vi "DSF.Execution.Builder.Build.vi"(8 "error in (no error)":errorcluster, 9 "Transfer ID":i32, 10 "Plugin ID":i32, 11 "Builder in":refnum<class "DSF.Execution.Builder.lvclass">) -> (0 "error out":errorcluster, 3 "Builder out":refnum<class "DSF.Execution.Builder.lvclass">)   [LabVIEW 2016, in "DSF.Engine.lvlib" / "DSF.Execution.Builder.lvclass"]
uses:
  DSF.Execution.Builder.lvclass
  DSF.Execution.Builder.lvclass/DSF.Execution.Builder.ctl
  Memory.Cache/DSF.Memory.Cache.Framework.lvclass/DSF.Memory.Cache.Framework.ctl
  Memory.Cache/DSF.Memory.Cache.Plugin.lvclass/DSF.Memory.Cache.Plugin.ctl
  Memory.Cache/DSF.Memory.Cache.Transfer.lvclass/DSF.Memory.Cache.Transfer.ctl
  Memory.Pointer/DSF.Memory.Pointer.VS Channels.lvclass/DSF.Memory.Pointer.VS Channels.ctl
  Submodules/Memory Manager/Source/Classes/Pointer/Memory.Pointer.lvclass/Memory.Pointer.ctl
  Memory.Buffer/Methods/DSF.Memory.Buffer.Write.vi
  Memory.Buffer/Methods/DSF.Memory.Buffer.Write.1D.Bool.vi
  Memory.Buffer/Methods/DSF.Memory.Buffer.Write.1D.SGL.vi
  Memory.Buffer/Methods/DSF.Memory.Buffer.Write.1D.DBL.vi
  Memory.Buffer/Methods/DSF.Memory.Buffer.Write.1D.I8.vi
  Memory.Buffer/Methods/DSF.Memory.Buffer.Write.1D.I16.vi
  Memory.Buffer/Methods/DSF.Memory.Buffer.Write.1D.I32.vi
  Memory.Buffer/Methods/DSF.Memory.Buffer.Write.1D.I64.vi
  Memory.Buffer/Methods/DSF.Memory.Buffer.Write.1D.U8.vi
  Memory.Buffer/Methods/DSF.Memory.Buffer.Write.1D.U16.vi
  Memory.Buffer/Methods/DSF.Memory.Buffer.Write.1D.U32.vi
  Memory.Buffer/Methods/DSF.Memory.Buffer.Write.1D.U64.vi
  Memory.Cache/DSF.Memory.Cache.Framework.Get Plugin Caches.vi
  Memory.Cache/DSF.Memory.Cache.Plugin.Get Transfer Caches.vi
  Memory.Pointer/DSF.Memory.Pointer.VS Channels.Get Channel Count.vi
  Submodules/Memory Manager/Source/Classes/Pointer/Methods/Memory.Pointer.Read.vi
  Submodules/Memory Manager/Source/Classes/Pointer/Methods/Memory.Pointer.Read.Safe.1D.DBL.vi
  Submodules/Memory Manager/Source/Classes/Pointer/Methods/Memory.Pointer.Write.vi
  Submodules/Memory Manager/Source/Classes/Pointer/Methods/Memory.Pointer.Write.Safe.1D.Bool.vi
  Submodules/Memory Manager/Source/Classes/Pointer/Methods/Memory.Pointer.Write.Safe.1D.SGL.vi
  Submodules/Memory Manager/Source/Classes/Pointer/Methods/Memory.Pointer.Write.Safe.1D.DBL.vi
  Submodules/Memory Manager/Source/Classes/Pointer/Methods/Memory.Pointer.Write.Safe.1D.I8.vi
  Submodules/Memory Manager/Source/Classes/Pointer/Methods/Memory.Pointer.Write.Safe.1D.I16.vi
  Submodules/Memory Manager/Source/Classes/Pointer/Methods/Memory.Pointer.Write.Safe.1D.I32.vi
  Submodules/Memory Manager/Source/Classes/Pointer/Methods/Memory.Pointer.Write.Safe.1D.I64.vi
  Submodules/Memory Manager/Source/Classes/Pointer/Methods/Memory.Pointer.Write.Safe.1D.U8.vi
  Submodules/Memory Manager/Source/Classes/Pointer/Methods/Memory.Pointer.Write.Safe.1D.U16.vi
  Submodules/Memory Manager/Source/Classes/Pointer/Methods/Memory.Pointer.Write.Safe.1D.U32.vi
  Submodules/Memory Manager/Source/Classes/Pointer/Methods/Memory.Pointer.Write.Safe.1D.U64.vi
  Submodules/Memory Manager/Source/Classes/Pointer/Methods/Memory.Pointer.Read.Unsafe.1D.DBL.vi
  Submodules/Memory Manager/Source/Classes/Pointer/Methods/Memory.Pointer.Parameter Check.Null Pointer.vi
  Submodules/Memory Manager/Source/Classes/Pointer/Methods/Memory.Pointer.Parameter Check.Subset.Power of 2.vi
  Submodules/Memory Manager/Source/Classes/Pointer/Methods/Memory.Pointer.Write.Unsafe.1D.Bool.vi
  Submodules/Memory Manager/Source/Classes/Pointer/Methods/Memory.Pointer.Write.Unsafe.1D.SGL.vi
  Submodules/Memory Manager/Source/Classes/Pointer/Methods/Memory.Pointer.Write.Unsafe.1D.DBL.vi
  Submodules/Memory Manager/Source/Classes/Pointer/Methods/Memory.Pointer.Write.Unsafe.1D.I8.vi
  Submodules/Memory Manager/Source/Classes/Pointer/Methods/Memory.Pointer.Write.Unsafe.1D.I16.vi
  Submodules/Memory Manager/Source/Classes/Pointer/Methods/Memory.Pointer.Write.Unsafe.1D.I32.vi
  Submodules/Memory Manager/Source/Classes/Pointer/Methods/Memory.Pointer.Write.Unsafe.1D.I64.vi
  Submodules/Memory Manager/Source/Classes/Pointer/Methods/Memory.Pointer.Write.Unsafe.1D.U8.vi
  Submodules/Memory Manager/Source/Classes/Pointer/Methods/Memory.Pointer.Write.Unsafe.1D.U16.vi
  Submodules/Memory Manager/Source/Classes/Pointer/Methods/Memory.Pointer.Write.Unsafe.1D.U32.vi
  Submodules/Memory Manager/Source/Classes/Pointer/Methods/Memory.Pointer.Write.Unsafe.1D.U64.vi
  Submodules/Memory Manager/Source/Classes/Pointer/Accessors/Get Address.vi
  Submodules/Memory Manager/Source/Classes/Pointer/Methods/Memory.Pointer.Errors.vi
  Submodules/Memory Manager/Source/Classes/Pointer/Methods/Memory.Pointer.Errors.Null Pointer.vi
  Submodules/Memory Manager/Source/Classes/Pointer/Methods/Memory.Pointer.Errors.Out of Bounds.vi
  Submodules/Memory Manager/Source/Classes/Pointer/Accessors/Get Size.vi
  Submodules/Memory Manager/Source/VIs/Memory.Count to Size.Power of 2.vi
  Submodules/Memory Manager/Source/Classes/Pointer/Methods/Memory.Pointer.Errors.Create Error.vi
  Submodules/Memory Manager/Source/Submodules/SEH/Source/VIs/Static Error Handling.Source Buffer.Write.String.vi
  Submodules/Memory Manager/Source/Classes/Pointer/Methods/Memory.Pointer.Errors.Write Pointer Size.vi
  Submodules/Memory Manager/Source/Submodules/SEH/Source/VIs/Static Error Handling.Source Buffer.Write.Numeric.Scalar.Base10.vi
  Submodules/Memory Manager/Source/Submodules/SEH/Source/VIs/Static Error Handling.Source Buffer.Write.Numeric.Scalar.Base10 (U64).vi
  Submodules/Memory Manager/Source/Submodules/SEH/Source/VIs/Static Error Handling.Error Cluster Constant.vi
  Submodules/Memory Manager/Source/Submodules/SEH/Source/VIs/Static Error Handling.Error Cluster Constant (256B).vi
  Submodules/Memory Manager/Source/Submodules/SEH/Source/VIs/Static Error Handling.Parameters.Status.Set.vi
  Submodules/Memory Manager/Source/Submodules/SEH/Source/VIs/Static Error Handling.Parameters.Code.Set.vi
  Submodules/Memory Manager/Source/Submodules/SEH/Source/VIs/Static Error Handling.Parameters.VI Source.Set.vi
  Submodules/Memory Manager/Source/Constants/Memory.Constants.vi
  Submodules/Memory Manager/Source/Constants/Memory.Constants.Library Name.vi
  Submodules/Memory Manager/Source/Classes/Pointer/Methods/Memory.Pointer.Errors.Get Info.vi
  Memory.Pointer/DSF.Memory.Pointer.VS Channels.lvclass
  C:/Git/SourceTree/DSF/Source/Submodules/Memory Manager/Source/Classes/Pointer/Memory.Pointer.lvclass
  Memory.Buffer/DSF.Memory.Buffer.lvclass
  Memory.Cache/DSF.Memory.Cache.Framework.lvclass
  Memory.Cache/DSF.Memory.Cache.Plugin.lvclass
  Memory.Cache/DSF.Memory.Cache.Transfer.lvclass
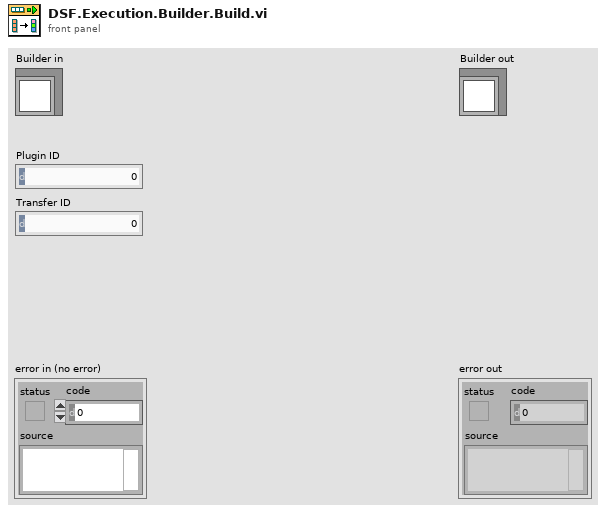
[diagram p1: front panel]
types:
  T1 = typedef "DSF.Memory.lvlib/DSF.Memory.Buffer Channel Configuration.ctl" = cluster{"data type":T2, "offset":u64, "count":u64, "index":u64}
  T2 = typedef "DSF.Shared.lvlib/DSF.Common.Data Type.ctl" = enum8{"Bool", "SGL", "DBL", "I8", "I16", "I32", "I64", "U8", "U16", "U32", "U64"}
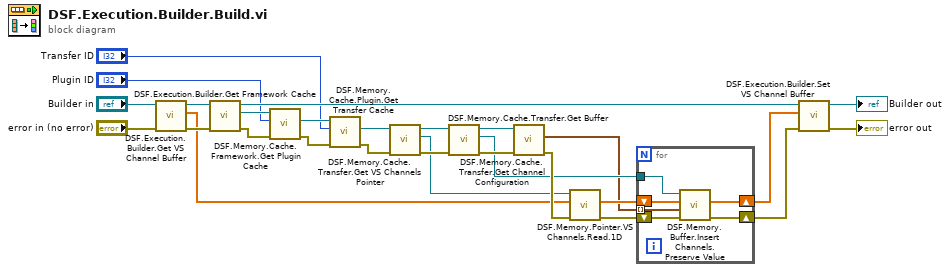
[diagram p0: block diagram]
diagram:
  n1 = call "DSF.Execution.Builder.Get VS Channel Buffer.vi"("error in (no error)"="error in (no error)", "Builder in"="Builder in") -> ("error out"=w15:errorcluster, "VS Channel Buffer"=w14:dbl[], "Builder out"=w16:refnum<class "DSF.Execution.Builder.lvclass">)  [unwired: 7 in]
  n2 = call "DSF.Execution.Builder.Get Framework Cache.vi"("error in (no error)"=w15, "Builder in"=w16) -> ("error out"=w20:errorcluster, "Framework Cache"=w23:refnum<class "DSF.Memory.Cache.Framework.lvclass">, "Builder out"=w5:refnum<class "DSF.Execution.Builder.lvclass">)  [unwired: 7 in]
  n3 = call "DSF.Memory.Cache.Framework.Get Plugin Cache.vi"("error in (no error)"=w20, "Plugin ID"="Plugin ID", "Framework Cache in"=w23) -> ("error out"=w21:errorcluster, "Plugin Cache"=w22:refnum<class "DSF.Memory.Cache.Plugin.lvclass">)  [unwired: 6 in, 1 out]
  n4 = call "DSF.Memory.Cache.Plugin.Get Transfer Cache.vi"("error in (no error)"=w21, "Transfer ID"="Transfer ID", "Plugin Cache in"=w22) -> ("error out"=w18:errorcluster, "Transfer Cache"=w19:refnum<class "DSF.Memory.Cache.Transfer.lvclass">)  [unwired: 6 in, 1 out]
  n5 = call "DSF.Memory.Cache.Transfer.Get VS Channels Pointer.vi"("error in (no error)"=w18, "Transfer Cache in"=w19) -> ("error out"=w9:errorcluster, "VS Channels Pointer"=w7:refnum<class "DSF.Memory.Pointer.VS Channels.lvclass">, "Transfer Cache out"=w10:refnum<class "DSF.Memory.Cache.Transfer.lvclass">)  [unwired: 7 in]
  n6 = call "DSF.Memory.Cache.Transfer.Get Buffer.vi"("error in (no error)"=w9, "Transfer Cache in"=w10) -> ("error out"=w8:errorcluster, "Buffer"=w6:refnum<class "DSF.Memory.Buffer.lvclass">, "Transfer Cache out"=w1:refnum<class "DSF.Memory.Cache.Transfer.lvclass">)  [unwired: 7 in]
  n7 = call "DSF.Memory.Cache.Transfer.Get Channel Configuration.vi"("error in (no error)"=w8, "Transfer Cache in"=w1) -> ("error out"=w24:errorcluster, "Channel Configuration"=w2:T1[])  [unwired: 7 in, 1 out]
  n8 = call "DSF.Memory.Pointer.VS Channels.Read.1D.vi"("error in (no error)"=w24, "Channels Array in"=w14, "VS Channels Pointer in"=w7) -> ("error out"=w12:errorcluster, "Channels Array out"=w17:dbl[])  [unwired: 5 in, 2 out]
  n9 = for {
    tunnel: w2 -> [w29] mode=indexing
    shift-right: [w32] -> w13
    shift-left: w17 -> [w33]
    shift-right: [w31] -> w11
    shift-left: w12 -> [w34]
    tunnel: w6 -> [w30]
    n10 = call "DSF.Memory.Buffer.Insert Channels.Preserve Value.vi"("error in (no error)"=w34, "Channel Configuration"=w29, "VS Channels Array in"=w33, "Buffer in"=w30) -> ("error out"=w31:errorcluster, "VS Channels Array out"=w32:dbl[])  [unwired: 5 in, 1 out]
  }
  n11 = call "DSF.Execution.Builder.Set VS Channel Buffer.vi"("error in (no error)"=w11, "VS Channel Buffer"=w13, "Builder in"=w5) -> ("error out"=→"error out":errorcluster, "Builder out"=→"Builder out":refnum<class "DSF.Execution.Builder.lvclass">)  [unwired: 7 in]
